vi "DC_CNTRL_enquire_current_module.vi"(8 "error in (no error)":errorcluster, 11 "Handle":u64) -> (0 "error out":errorcluster, 1 "Module Type":string, 2 "Module number":i32, 3 "Handle out":u64)   [LabVIEW 2019]
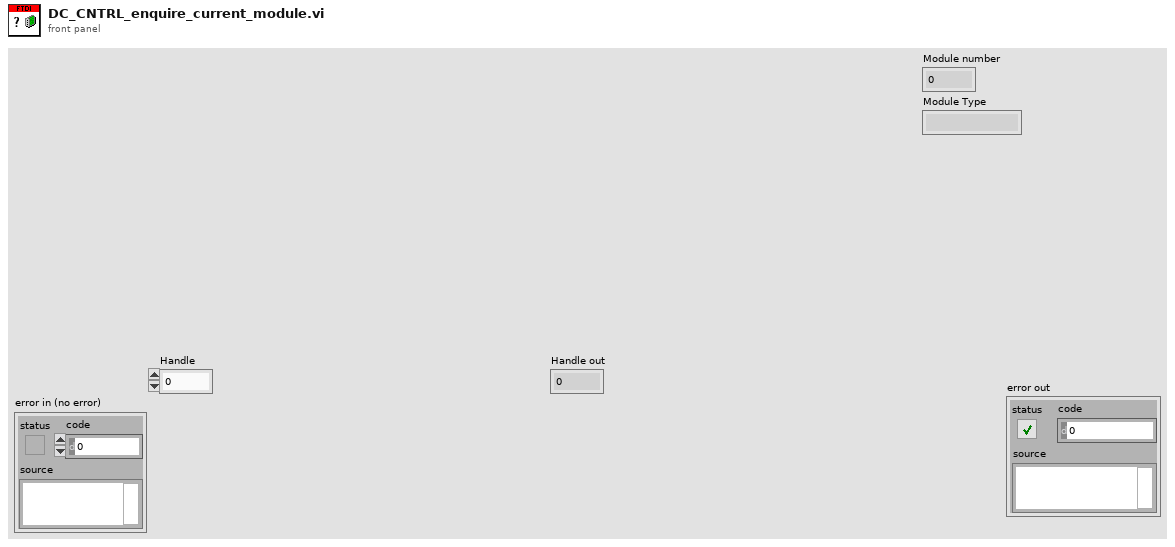
[diagram p1: front panel]
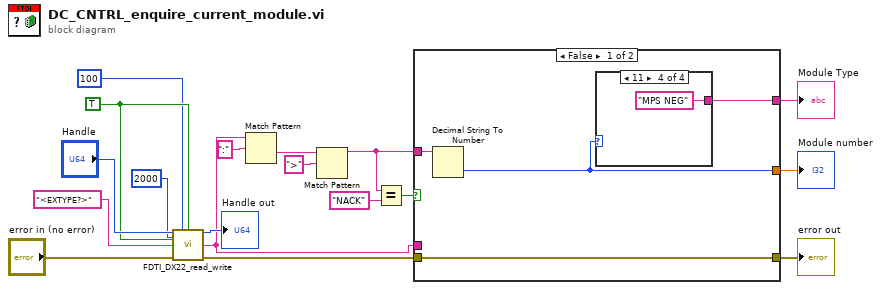
[diagram p0: block diagram]
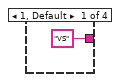
[diagram p2: hidden frame]
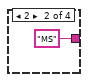
[diagram p3: hidden frame]
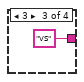
[diagram p4: hidden frame]
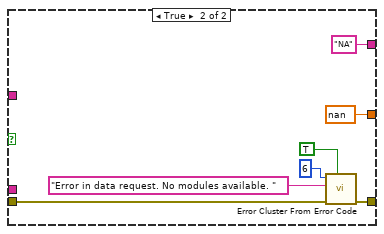
[diagram p5: hidden frame]
diagram:
  w13 = TRUE ("Clear  RxTx Buffer?")
  n1 = call "FDTI_DX22_read_write.vi"("Handle"="Handle", "Bytes to wait for"=100, "Read Answer?"=w13, "Bytes wait timeout / ms"=2000, "Clear  RxTx Buffer?"=w13, "Write string"="<EXTYPE?>" ("string"), "error in (no error)"="error in (no error)") -> ("Handle out"=→"Handle out":u64, "Read Data"=w6:string, "error out"=w7:errorcluster)  [unwired: 6 in]
  n2 = Match Pattern(string=w6, regular expression=":") -> (after substring=w11:string)  [unwired: 1 in, 3 out]
  n3 = Match Pattern(string=w11, regular expression=">") -> (before substring=w3:string)  [unwired: 1 in, 3 out]
  n4 = Equal?(x=w3, y="NACK") -> (x = y?=w9:bool)
  n5 = case shown="False" w9 {
    tunnel: w7 -> [w22 w33]
    tunnel: w6 -> [_ _]
    tunnel: [w22 w29] -> w5
    tunnel: w3 -> [w21 _]
    tunnel: [w20 "NA"] -> w1
    tunnel: [w19 nan] -> w2
    frame False {
      n6 = Decimal String To Number(string=w21) -> (number=w19:i32)  [unwired: 2 in, 1 out]
      n7 = case shown="11" w19 {
        tunnel: ["VS" "MS" "VS" "MPS NEG"] -> w20
        frame 1, Default {
        }
        frame 2 {
        }
        frame 3 {
        }
        frame 11 {
        }
      }
    }
    frame True {
      n8 = call <vilib>:"Error Cluster From Error Code.vi"("show call chain? (False)"=TRUE, "error in (no error)"=w33, "error message (\"\")"="Error in data request. No modules available. " ("error message (\"\")"), "error code (0)"=6) -> ("error out"=w29:errorcluster)  [unwired: 5 in]
    }
  }
  "error out" <- w5
  "Module number" <- w2
  "Module Type" <- w1
